vi "release_hw.vi"(8 "error in (no error)":errorcluster, 11 "stresing in":refnum<class "stresing.lvclass">) -> (0 "error out":errorcluster, 3 "stresing out":refnum<class "stresing.lvclass">)   [LabVIEW 2019, in "stresing.lvlib" / "stresing.lvclass"]
uses:
  stresing.lvclass
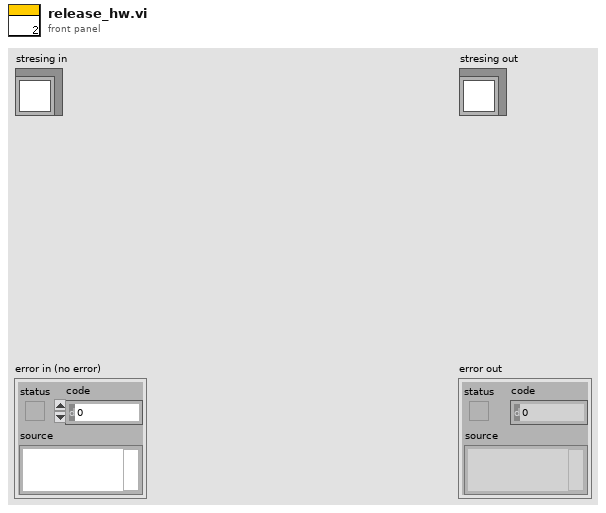
[diagram p1: front panel]
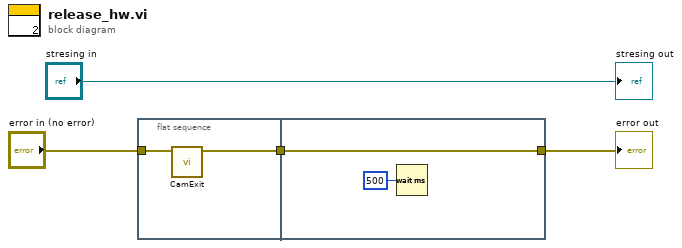
[diagram p0: block diagram]
diagram:
  n1 = flat-sequence {
    tunnel: "error in (no error)" -> [w6]
    tunnel: [w5] -> w3
    tunnel: w3 -> [w7]
    tunnel: [w7] -> w2
    frame #0 {
      n2 = call "CamExit.vi"("Camera error in"=w6) -> ("Camera error out"=w5:errorcluster)  [unwired: 10 in]
    }
    frame #1 {
      n3 = Wait (ms)(milliseconds to wait=u32 500) -> ()  [unwired: 1 out]
    }
  }
  "error out" <- w2
  "stresing out" <- "stresing in"
